vi "chipKIT Max32.vi"() -> (0 "chipKIT Max32":T1={"DI Channels"=[0, 1, 2, 3, 4, 5, 6, 7, 8, 9, 10, 11, 12, 13, 22, 23, 24, 25, 26, 27, 28, 29, 30, 31, 32, 33, 34, 35, 36, 37, 38, 39, 40, 41, 42, 43, 44, 45, 46, 47, 48, 49, 50, 51, 52, 53, 70, 71, 72, 73, 74, 75, 76, 77, 78, 79, 80, 81, 82, 83, 84, 85], "DO Channels"=[0, 1, 2, 3, 4, 5, 6, 7, 8, 9, 10, 11, 12, 13, 22, 23, 24, 25, 26, 27, 28, 29, 30, 31, 32, 33, 34, 35, 36, 37], "AI"=[0, 1, 2, 3, 4, 5, 6, 7, 8, 9, 10, 11, 12, 13, 14, 15], "AO"=[], "PWM"=[3, 5, 6, 9, 10], "QE"=[], "UART"=[0, 1, 2, 3], "I2C 2"=[0], "SPI"=[0], "CAN"=[0, 1], "AI Ref (V)"=3.3, "Firmware Program Interfaces"=[enum."Serial / USB"], "Firmware Versions"=[{"Name"="LINX - Serial Interface", "Relative Path"="\\Digilent\\chipKIT\\Max32\\Max32_Serial_USB.hex ", "Firmware Interface"=enum."Serial "}, {"Name"="LINX - Ethernet Interface", "Relative Path"="\\Digilent\\chipKIT\\Max32\\Max32_Ethernet.hex ", "Firmware Interface"=enum."Ethernet"}, {"Name"="LINX - Serial Interface [DEBUG]", "Relative Path"="\\Digilent\\chipKIT\\Max32\\Max32_Serial_USB_Debug.hex ", "Firmware Interface"=enum."Serial "}, {"Name"="LINX - Ethernet Interface [DEBUG]", "Relative Path"="\\Digilent\\chipKIT\\Max32\\Max32_Ethernet_Debug.hex ", "Firmware Interface"=enum."Ethernet"}], "Name"="chipkit Max32", "AO Resolution (Bits)"=0, "AO Ref (V)"=0.0})   [LabVIEW 2011, in "LMH-LINX.lvlib"]
doc: "I/O description of the chipKIT Max32."
uses:
  LMH-LINX.lvlib
  Generic Device.ctl
  Firmware Version.ctl
  Device/Type Defs/Firmware Interface.ctl
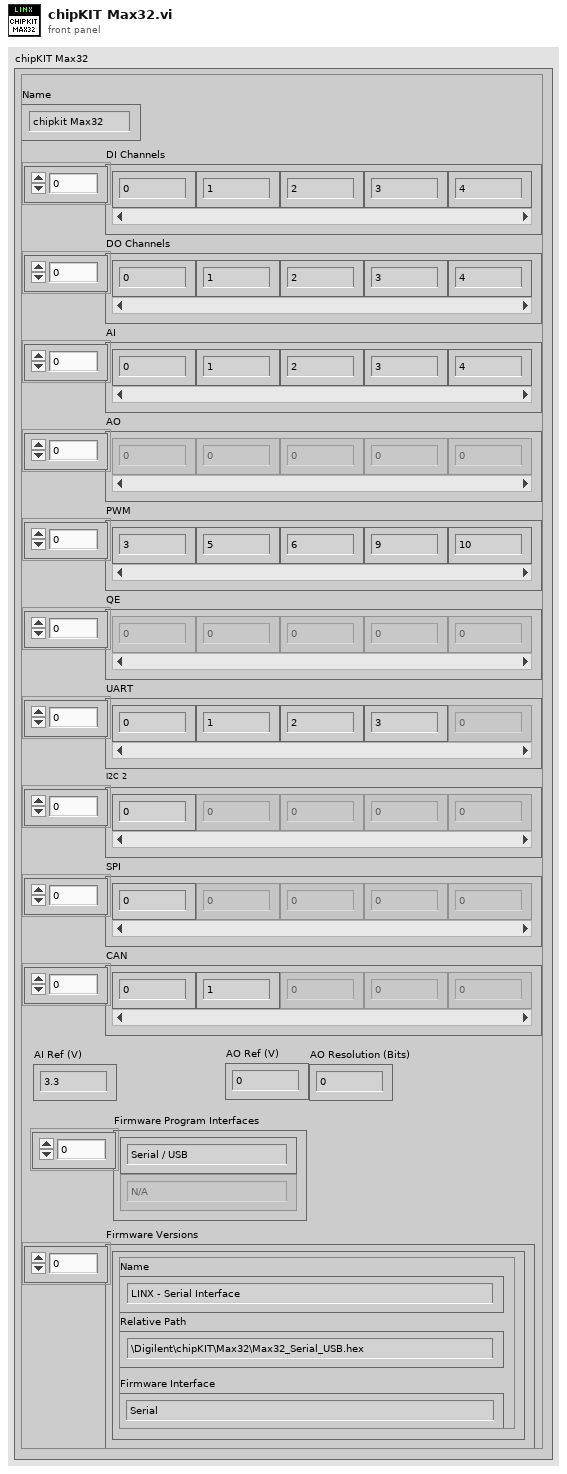
[diagram p1: front panel]
types:
  T1 = typedef "LMH-LINX.lvlib/Generic Device.ctl" = cluster{"DI Channels":u8[], "DO Channels":u8[], "AI":u8[], "AO":u8[], "PWM":u8[], "QE":u8[], "UART":u8[], "I2C 2":u8[], "SPI":u8[], "CAN":u8[], "AI Ref (V)":dbl, "Firmware Program Interfaces":enum16{"N/A", "Serial / USB", "USB", "TCP"}[], "Firmware Versions":T2[], "Name":string, "AO Resolution (Bits)":u8, "AO Ref (V)":dbl}
  T2 = typedef "LMH-LINX.lvlib/Firmware Version.ctl" = cluster{"Name":string, "Relative Path":string, "Firmware Interface":T3}
  T3 = typedef "LMH-LINX.lvlib/Firmware Interface.ctl" = enum32{"Serial ", "Ethernet", "WIFI"}
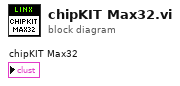
[diagram p0: block diagram]
diagram:
